vi "test.vi"() -> ()   [LabVIEW 2017]
uses:
  sql_LV_plus.llb/sql_insert.vi
  sql_LV_plus.llb/sql_select.vi
  sql_LV_plus.llb/sql_cmd.vi
  sql_LV_plus.llb/sql_update.vi
  sql_LV_plus.llb/sql_tables.vi
  sql_LV_plus.llb/sql_columns.vi
  sql_LV_plus.llb/sql_delete.vi
  sql_LV_plus.llb/sql_XML.vi
panel:
  out "SQL results":string[][](array[string])
  out "col_headers":string[](array[string])
  out "results":cluster{"idx":i32, "data":dbl}[](array[cluster]) {"data" format="%.2f"}
  in  "db":T1={"db"="", "host"="test_db", "user"="danny", "password"="danny", "db_type"=enum."odbc"}
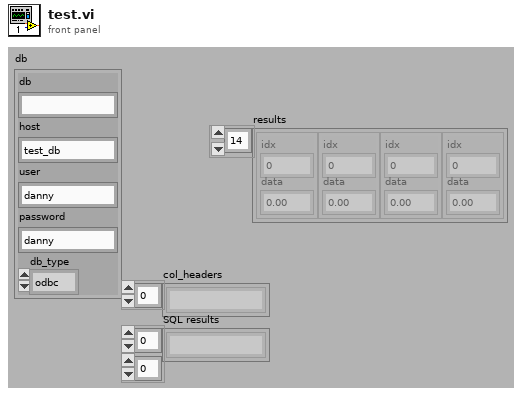
[diagram p1: front panel]
types:
  T1 = cluster{"db":string, "host":string, "user":string, "password":string, "db_type":enum16{"mysql", "odbc"}}
  T2 = cluster{"idx":i32, "voltage":dbl, "temperature":dbl}[]
  T3 = enum16{"MySQL", "Oracle", "DB2", "FireBird", "MS Access", "SQL Server", "PostgreSQL"}
  T4 = cluster{"idx":i32, "voltage":dbl, "temperature":dbl}
  T5 = cluster{"idx":i32, "data":dbl, "data2 + data3":dbl}
  T6 = cluster{"temp.idx":i32, "temp.data":dbl, "temp.data2 + swept_data.data3":dbl}
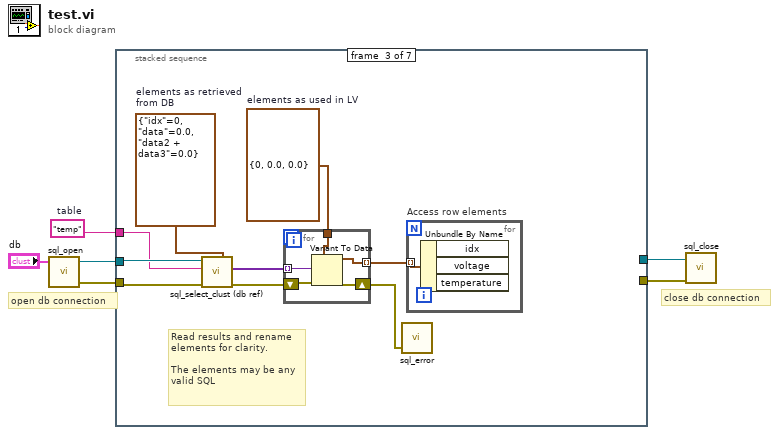
[diagram p0: block diagram]
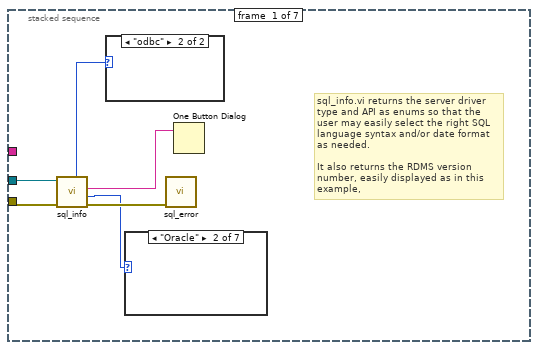
[diagram p2: hidden frame]
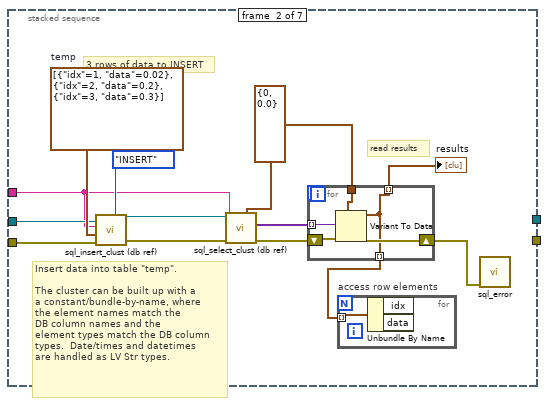
[diagram p10: hidden frame]
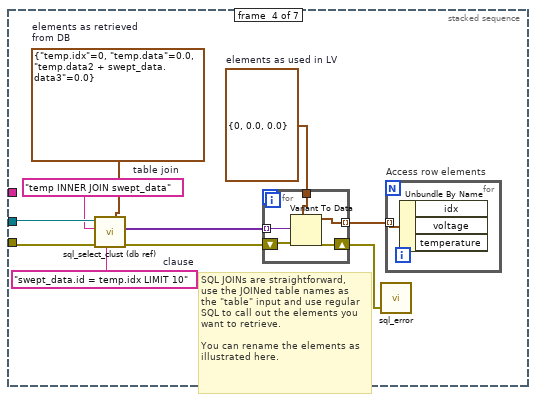
[diagram p11: hidden frame]
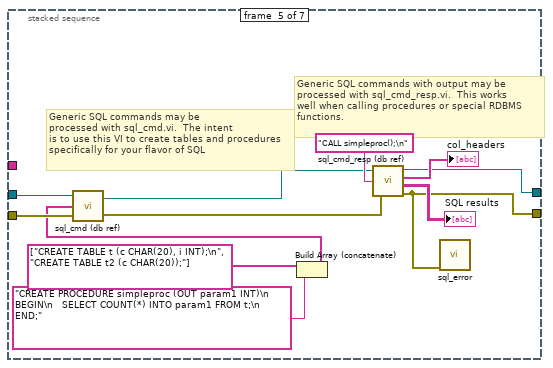
[diagram p12: hidden frame]
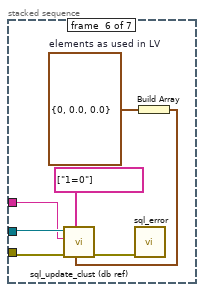
[diagram p13: hidden frame]
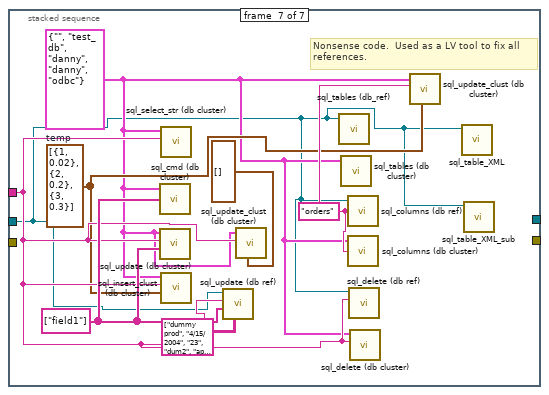
[diagram p14: hidden frame]
diagram:
  w1 = "temp"  # table
  # "close db connection"
  # "open db connection"
  n1 = call "sql_open.vi"("db"="db") -> ("error out"=w4:errorcluster, "refnum"=w5:refnum<vi>)  [unwired: 2 in, 1 out]
  n2 = stacked-sequence {
    tunnel: w5 -> [w12 w17 w37 w53 w66 w81 w82]
    tunnel: w4 -> [w11 w16 w36 w52 w74 w76 _]
    tunnel: [_ _ _ _ w63 _ _] -> w3
    tunnel: [_ _ _ _ w64 _ _] -> w2
    tunnel: w1 -> [_ w14 w34 _ _ w80 w86]
    frame #0 {
      # "sql_info.vi returns the server driver\ntype and API as enums so that the user may easily select the right SQL language syntax and/or date format as needed.\n\nIt also returns the RDMS version number, easily displayed as in this example,"
      n3 = call "sql_info.vi"("error in"=w11, "refnnum"=w12) -> ("error out"=w10:errorcluster, "driver"=w9:T3, "info string"=w8:string, "db_type"=w7:enum16{"mysql", "odbc"})  [unwired: 3 in, 1 out]
      n4 = case shown="\"odbc\"" w7 {
        frame "mysql", Default {
        }
        frame "odbc" {
        }
      }
      n5 = case shown="\"Oracle\"" w9 {
        frame "MySQL", Default {
        }
        frame "Oracle" {
        }
        frame "DB2" {
        }
        frame "FireBird" {
        }
        frame "MS Access" {
        }
        frame "SQL Server" {
        }
        frame "PostgreSQL" {
        }
      }
      n6 = call "sql_error.vi"("error in (no error)"=w10) -> ()  [unwired: 10 in, 1 out]
      n7 = One Button Dialog(message=w8) -> ()  [unwired: 1 in, 1 out]
    }
    frame #1 {
      w23 = cluster{"idx":i32, "data":dbl} {"idx"=0, "data"=0.0}
      w25 = cluster{"idx":i32, "data":dbl}[] [{"idx"=1, "data"=0.02}, {"idx"=2, "data"=0.2}, {"idx"=3, "data"=0.3}]  # temp
      # "3 rows of data to INSERT"
      # "read results"
      # "Insert data into table \"temp\".\n\nThe cluster can be built up with a\na constant/bundle-by-name, where\nthe element names match the \nDB column names and the\nelement types match the DB column\ntypes.  Date/times and datetimes\nare handled as LV Str types."
      n8 = call-poly "sql_insert_clust (db ref).vi"("operation"=enum16{"INSERT", "REPLACE"}."INSERT", "error in"=w16, "data in"=w25, "table"=w14, "refnum"=w17) -> ("error out"=w21:errorcluster, "dup refnum"=w22:refnum<vi>)  [unwired: 4 in, 1 out]
      n9 = call-poly "sql_select_clust (db ref).vi"("type"=w23, "error in"=w21, "table"=w14, "refnum"=w22) -> ("error out"=w20:errorcluster, "Values"=w19:variant[])  [unwired: 5 in, 1 out]
      n10 = for {
        shift-right: [w31] -> w13
        shift-left: w20 -> [w30]
        tunnel: w19 -> [w29] mode=indexing
        tunnel: w23 -> [w28]
        tunnel: [w27] -> w18 mode=indexing
        tunnel: [w27] -> w15 mode=indexing
        n11 = Variant To Data(error in=w30, type=w28, Variant=w29) -> (data=w27:cluster{"idx":i32, "data":dbl}, error out=w31:errorcluster)
      }
      "results" <- w18
      n12 = for "access row elements" {
        tunnel: w15 -> [w26] mode=indexing
        n13 = Unbundle By Name(w26) -> ()  [unwired: 2 out]
      }
      n14 = call "sql_error.vi"("error in (no error)"=w13) -> ()  [unwired: 10 in, 1 out]
    }
    frame #2 {
      w35 = T4 {"idx"=0, "voltage"=0.0, "temperature"=0.0}  # elements as used in LV
      w38 = T5 {"idx"=0, "data"=0.0, "data2 + data3"=0.0}  # elements as retrieved from DB
      # "Read results and rename\nelements for clarity.\n\nThe elements may be any\nvalid SQL"
      n15 = call-poly "sql_select_clust (db ref).vi"("type"=w38, "error in"=w36, "table"=w34, "refnum"=w37) -> ("error out"=w40:errorcluster, "Values"=w39:variant[])  [unwired: 5 in, 1 out]
      n16 = for {
        shift-right: [w46] -> w32
        shift-left: w40 -> [w45]
        tunnel: w39 -> [w44] mode=indexing
        tunnel: w35 -> [w43]
        tunnel: [w42] -> w33 mode=indexing
        n17 = Variant To Data(error in=w45, type=w43, Variant=w44) -> (data=w42:T4, error out=w46:errorcluster)
      }
      n18 = call "sql_error.vi"("error in (no error)"=w32) -> ()  [unwired: 10 in, 1 out]
      n19 = for "Access row elements" {
        tunnel: w33 -> [w41] mode=indexing
        n20 = Unbundle By Name(w41) -> ()  [unwired: 3 out]
      }
    }
    frame #3 {
      w47 = "swept_data.id = temp.idx LIMIT 10"  # clause
      w48 = "temp INNER JOIN swept_data"  # table join
      w51 = T4 {"idx"=0, "voltage"=0.0, "temperature"=0.0}  # elements as used in LV
      w54 = T6 {"temp.idx"=0, "temp.data"=0.0, "temp.data2 + swept_data.data3"=0.0}  # elements as retrieved from DB
      # "SQL JOINs are straightforward,\nuse the JOINed table names as\nthe \"table\" input and use regular\nSQL to call out the elements you\nwant to retrieve.\n\nYou can rename the elements as\nillustrated here."
      n21 = call-poly "sql_select_clust (db ref).vi"("type"=w54, "clause"=w47, "error in"=w52, "table"=w48, "refnum"=w53) -> ("error out"=w56:errorcluster, "Values"=w55:variant[])  [unwired: 4 in, 1 out]
      n22 = for {
        shift-right: [w62] -> w49
        shift-left: w56 -> [w61]
        tunnel: w55 -> [w60] mode=indexing
        tunnel: w51 -> [w59]
        tunnel: [w58] -> w50 mode=indexing
        n23 = Variant To Data(error in=w61, type=w59, Variant=w60) -> (data=w58:T4, error out=w62:errorcluster)
      }
      n24 = call "sql_error.vi"("error in (no error)"=w49) -> ()  [unwired: 10 in, 1 out]
      n25 = for "Access row elements" {
        tunnel: w50 -> [w57] mode=indexing
        n26 = Unbundle By Name(w57) -> ()  [unwired: 3 out]
      }
    }
    frame #4 {
      # "Generic SQL commands with output may be\nprocessed with sql_cmd_resp.vi.  This works\nwell when calling procedures or special RDBMS\nfunctions."
      # "Generic SQL commands may be\nprocessed with sql_cmd.vi.  The intent\nis to use this VI to create tables and procedures\nspecifically for your flavor of SQL"
      n27 = Build Array (concatenate)(string[] ["CREATE TABLE t (c CHAR(20), i INT);\n", "CREATE TABLE t2 (c CHAR(20));"] ("sql_cmds"), "CREATE PROCEDURE simpleproc (OUT param1 INT)\n BEGIN\n   SELECT COUNT(*) INTO param1 FROM t;\n END;" ("where")) -> (w72:string[])
      n28 = call-poly "sql_cmd (db ref).vi"("error in"=w74, "sql_cmds"=w72, "refnum"=w66) -> ("error out"=w70:errorcluster, "dup refnum"=w65:refnum<vi>)
      n29 = call "sql_cmd_resp (db ref).vi"("refnum"=w65, "sql_cmd"="CALL simpleproc();\n" ("where"), "error in"=w70) -> ("dup refnum"=w64:refnum<vi>, "col_headers"=→"col_headers":string[], "results"=→"SQL results":string[][], "error out"=w63:errorcluster)
      n30 = call "sql_error.vi"("error in (no error)"=w63) -> ()  [unwired: 10 in, 1 out]
    }
    frame #5 {
      w79 = T4 {"idx"=0, "voltage"=0.0, "temperature"=0.0}  # elements as used in LV
      n31 = Build Array(w79) -> (w78:T2)
      n32 = call-poly "sql_update_clust (db ref).vi"("data in"=w78, "where"=string[] ["1=0"], "error in"=w76, "table"=w80, "refnum"=w81) -> ("error out"=w75:errorcluster)  [unwired: 4 in, 2 out]
      n33 = call "sql_error.vi"("error in (no error)"=w75) -> ()  [unwired: 10 in, 1 out]
    }
    frame #6 {
      w85 = "orders" ("table")
      w84 = cluster{"idx":i32, "data":dbl}[] [{"idx"=1, "data"=0.02}, {"idx"=2, "data"=0.2}, {"idx"=3, "data"=0.3}]  # temp
      w88 = string[] ["field1"] ("fields")
      w83 = T1 {"db"="", "host"="test_db", "user"="danny", "password"="danny", "db_type"=enum."odbc"} ("db")
      # "Nonsense code.  Used as a LV tool to fix all\nreferences."
      n34 = call-poly "sql_cmd (db cluster).vi"("sql_cmds"=w88, "db"=w83) -> ()  [unwired: 2 in, 1 out]
      n35 = call-poly "sql_update (db cluster).vi"("fields"=w88, "table"=w86, "db"=w83) -> ()  [unwired: 7 in, 2 out]
      n36 = call-poly "sql_select_str (db cluster).vi"("table"=w86, "db"=w83) -> ()  [unwired: 8 in, 2 out]
      n37 = call-poly "sql_insert_clust (db cluster).vi"("data in"=w84, "table"=w86, "db"=w83) -> ()  [unwired: 7 in, 2 out]
      n38 = call-poly "sql_update (db ref).vi"("values"=string[][] [["dummy prod", "4/15/2004", "23"], ["dum2", "april 15, 2004", "99"]], "fields"=w88, "table"=w86, "refnum"=w82) -> ()  [unwired: 5 in, 3 out]
      n39 = call-poly "sql_update_clust (db cluster).vi"("data in"=T2 [] ("appended array"), "table"=w86, "db"=w83) -> ()  [unwired: 7 in, 2 out]
      n40 = call-poly "sql_tables (db_ref).vi"("refnum"=w82) -> ()  [unwired: 2 in, 3 out]
      n41 = call-poly "sql_tables (db cluster).vi"("db"=w83) -> ()  [unwired: 3 in, 2 out]
      n42 = call-poly "sql_columns (db ref).vi"("table"=w85, "refnum"=w82) -> ()  [unwired: 1 in, 3 out]
      n43 = call-poly "sql_columns (db cluster).vi"("table"=w85, "db"=w83) -> ()  [unwired: 1 in, 3 out]
      n44 = call-poly "sql_delete (db ref).vi"("table"=w86, "refnum"=w82) -> ()  [unwired: 7 in, 3 out]
      n45 = call-poly "sql_delete (db cluster).vi"("table"=w86, "db"=w83) -> ()  [unwired: 8 in, 2 out]
      n46 = call-poly "sql_update_clust (db cluster).vi"("data in"=w84, "table"=w85, "db"=w83) -> ()  [unwired: 7 in, 2 out]
      n47 = call-poly "sql_table_XML.vi"("refnum"=w82) -> ()  [unwired: 8 in, 3 out]
      n48 = call-poly "sql_table_XML_sub.vi"("refnum"=w82) -> ()  [unwired: 8 in, 3 out]
    }
  }
  n49 = call "sql_close.vi"("error in"=w3, "refnum"=w2) -> ()  [unwired: 1 in, 1 out]
